vi "find_newest_file.vi"(7 "error in":errorcluster, 10 "Directory Path to Start the Search":path=path "C:/Program Files/National Instruments/LabVIEW 7.0") -> (0 "error out":errorcluster, 1 "List of All the File Names":string[](array[string]), 3 "Most Recent File Path":path)   [LabVIEW 2013]
doc: "This program finds all the files in a specified directory and then compares the last modified date and time for each file to find the most recently modified file. The for loop passes the index of the most current file and the array of file paths is indexed to get the file path of the most current file in the directory."
panel:
  # "- Select the directory path to start the search\n- Run the VI\n- The most recent file in the directory is displayed\n- List of All the File Names array contains the first-level files in the directory"
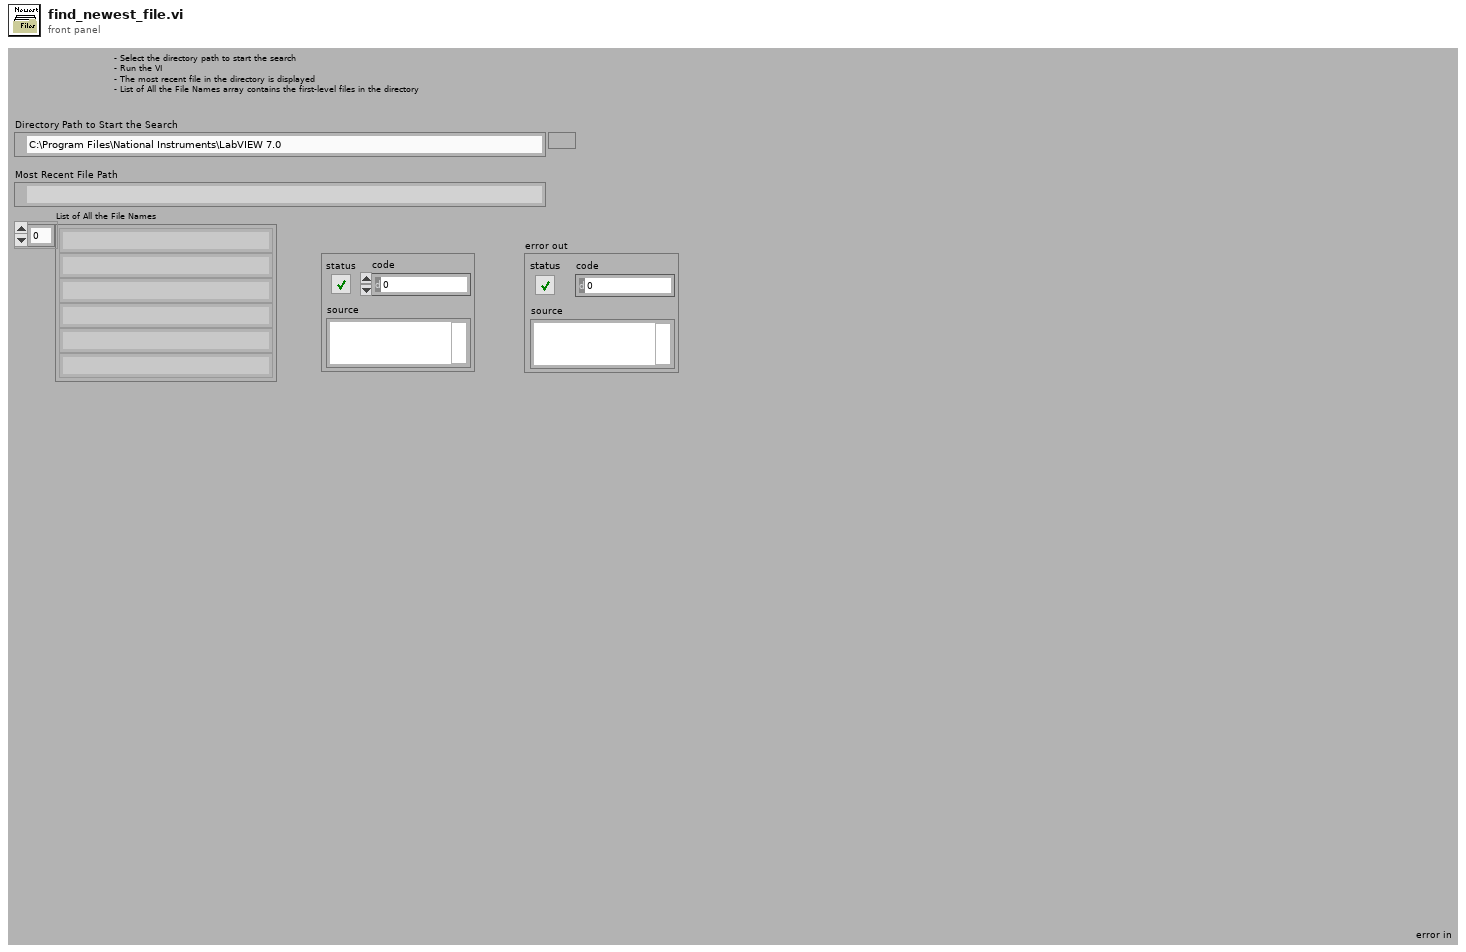
[diagram p1: front panel]
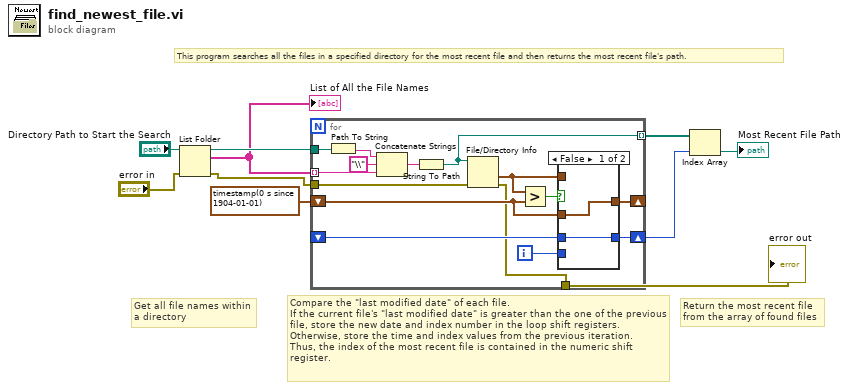
[diagram p0: block diagram]
diagram:
  # "Return the most recent file from the array of found files"
  # "Compare the \"last modified date\" of each file. \nIf the current file's \"last modified date\" is greater than the one of the previous file, store the new date and index number in the loop shift registers. \nOtherwise, store the time and index values from the previous iteration.\nThus, the index of the most recent file is contained in the numeric shift register."
  # "This program searches all the files in a specified directory for the most recent file and then returns the most recent file's path."
  # "Get all file names within a directory"
  n1 = List Folder(path="Directory Path to Start the Search", error in="error in") -> (path out=w10:path, filenames=w9:string[], error out=w2:errorcluster)  [unwired: 2 in, 1 out]
  "List of All the File Names" <- w9
  n2 = for {
    tunnel: w10 -> [w25]
    tunnel: w9 -> [w22] mode=indexing
    tunnel: [w20] -> w7 mode=indexing
    shift-right: [w15] -> _
    shift-left: timestamp(0 s since 1904-01-01) ("last mod") -> [w13]
    shift-right: [w17] -> w5
    shift-left: _ -> [w16]
    tunnel: w2 -> [w12]
    tunnel: [w11] -> w1
    i -> [w18]
    n3 = Path To String(path=w25) -> (string=w24:string)
    n4 = Concatenate Strings(w24, "\\" ("string"), w22) -> (w23:string)
    n5 = String To Path(string=w23) -> (path=w20:path)
    n6 = File/Directory Info(path=w20, error in=w12) -> (last mod=w14:timestamp, error out=w11:errorcluster)  [unwired: 5 out]
    n7 = Greater?(x=w14, y=w13) -> (0:w19:bool)
    n8 = case shown="False" w19 {
      tunnel: w14 -> [_ w29]
      tunnel: [w26 w29] -> w15
      tunnel: w18 -> [_ w28]
      tunnel: w13 -> [w26 _]
      tunnel: [w27 w28] -> w17
      tunnel: w16 -> [w27 _]
      frame False {
      }
      frame True {
      }
    }
  }
  "error out" <- w1
  n9 = Index Array(array=w7, index=w5) -> (element=→"Most Recent File Path":path)
